vi "Flush.vi"(8 "error in (no error)":errorcluster, 11 "Message Queue in":refnum<class "Message Queue.lvclass">) -> (0 "error out":errorcluster, 3 "Message Queue out":refnum<class "Message Queue.lvclass">)   [LabVIEW 2027, in "Messaging.lvlib" / "Message Queue.lvclass"]
uses:
  Message Queue.lvclass
  Message Queue.lvclass/Message Queue.ctl
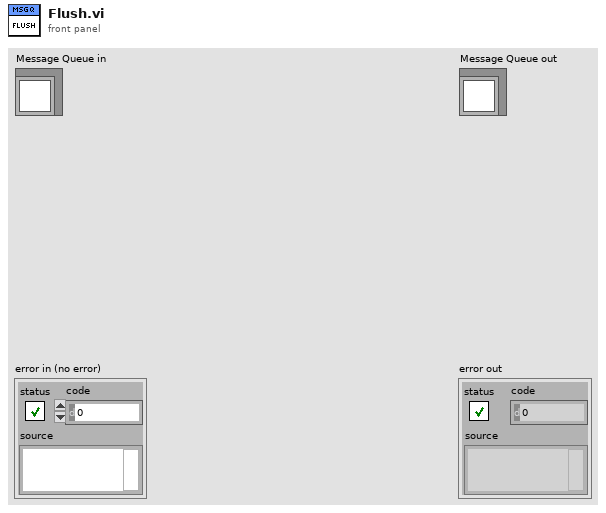
[diagram p1: front panel]
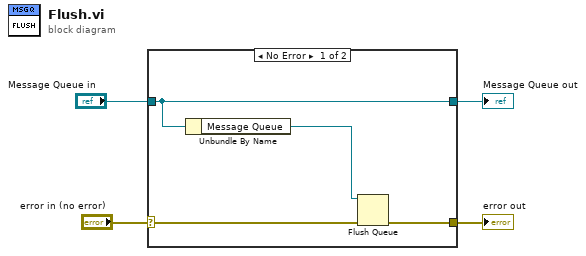
[diagram p0: block diagram]
diagram:
  n1 = case shown="No Error" "error in (no error)" {
    selector: "error in (no error)" -> [w8 w10]
    tunnel: [w7 w10] -> w3
    tunnel: [w6 w9] -> w2
    tunnel: "Message Queue in" -> [w6 w9]
    frame No Error {
      n2 = Unbundle By Name(w6) -> ("Message Queue"=w5:refnum<queue>)
      n3 = Flush Queue(queue=w5, error in (no error)=w8) -> (error out=w7:errorcluster)  [unwired: 2 out]
    }
    frame Error {
    }
  }
  "error out" <- w3
  "Message Queue out" <- w2
